vi "UI Post-Build Action.vi"(5 "Files Generated by Build":path[](array[path]), 6 "Top Level/Always Included VIs":path[](array[path]), 7 "Destination Path":path, 8 "error in (no error)":errorcluster, 9 "Target Name":string, 10 "Build Specification Name":string, 11 "Project Path":path) -> (0 "error out":errorcluster)   [LabVIEW 2021, in "CIF Build Actions.lvlib"]
uses:
  CIF Build Actions.lvlib
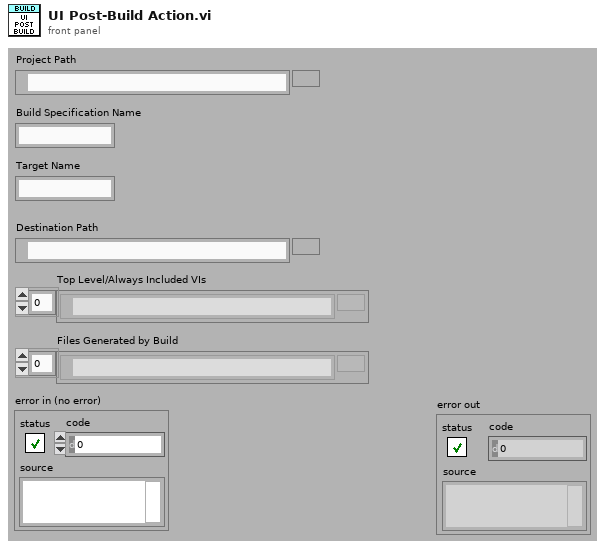
[diagram p1: front panel]
types:
  T1 = cluster{"Major":u16, "Minor":u16, "Fix":u16, "Build":u16}
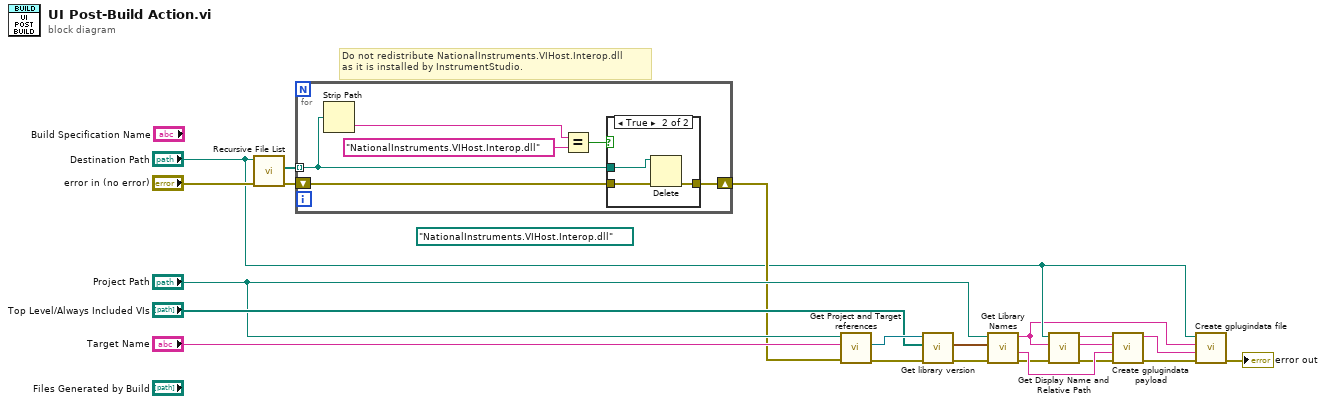
[diagram p0: block diagram]
diagram:
  (unwired) path "NationalInstruments.VIHost.Interop.dll" ("name or relative path")
  # "Do not redistribute NationalInstruments.VIHost.Interop.dll \nas it is installed by InstrumentStudio."
  n1 = call <vilib>:"Recursive File List.vi"("error in (no error)"="error in (no error)", "Folder Path"="Destination Path") -> ("error out"=w19:errorcluster, "All Files in Dir"=w20:path[])  [unwired: 5 in, 3 out]
  n2 = for {
    tunnel: w20 -> [w24] mode=indexing
    shift-right: [w22] -> w6
    shift-left: w19 -> [w23]
    n3 = Strip Path(path=w24) -> (name=w27:string)  [unwired: 1 out]
    n4 = Equal?(x=w27, y="NationalInstruments.VIHost.Interop.dll") -> (x = y?=w25:bool)
    n5 = case shown="True" w25 {
      tunnel: w24 -> [_ w31]
      tunnel: w23 -> [w28 w30]
      tunnel: [w28 w29] -> w22
      frame False {
      }
      frame True {
        n6 = Delete(path (use dialog)=w31, error in=w30) -> (error out=w29:errorcluster)  [unwired: 3 in, 2 out]
      }
    }
  }
  n7 = call "Get Project and Target references.vi"("error in (no error)"=w6, "Target Name"="Target Name", "Project Path"="Project Path") -> ("error out"=w13:errorcluster, "Target refnum"=w18:refnum<vi>)  [unwired: 6 in, 1 out]
  n8 = call "Get library version.vi"("error in (no error)"=w13, "Top Level/Always Included VIs"="Top Level/Always Included VIs", "Target reference in"=w18) -> ("error out"=w11:errorcluster, "Version"=w12:T1)  [unwired: 4 in, 3 out]
  n9 = call "Get Library Names.vi"("error in (no error)"=w11, "Version"=w12, "Project Path"="Project Path") -> ("error out"=w8:errorcluster, "Versioned Library (no extension)"=w9:string, "Library"=w2:string)  [unwired: 5 in, 1 out]
  n10 = call "Get Display Name and Relative Path.vi"("error in (no error)"=w8, "Library"=w2, "Destination Path"="Destination Path") -> ("error out"=w7:errorcluster, "Relative Path"=w15:string, "Display Name"=w14:string)  [unwired: 6 in]
  n11 = call "Create gplugindata payload.vi"("error in"=w7, "Library name with version"=w9, "Relative Path"=w15, "Display Name"=w14) -> ("error out"=w5:errorcluster, "gplugindata"=w4:string)  [unwired: 6 in]
  n12 = call "Create gplugindata file.vi"("error in"=w5, "gplugindata in"=w4, "Library"=w2, "Destination Path"="Destination Path") -> ("error out"=→"error out":errorcluster)  [unwired: 7 in]
